vi "While循环的先检查后执行.vi"() -> ()   [LabVIEW 2010]
panel:
  out "温度报警 2":bool
  in  "温度值":dbl(slide) scale=-10.0..10.0
  out "温度报警":bool
  in  "温度值":dbl(slide) scale=-10.0..10.0
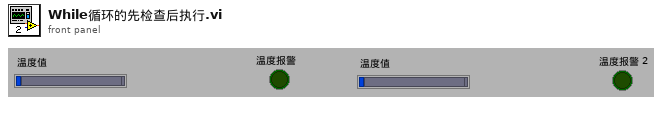
[diagram p1: front panel]
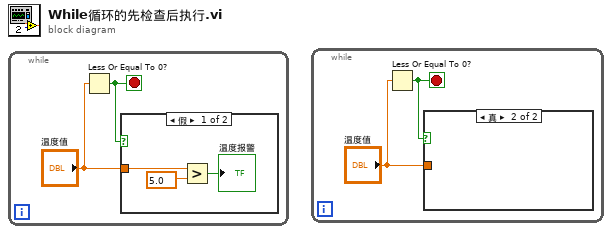
[diagram p0: block diagram]
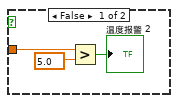
[diagram p2: hidden frame]
diagram:
  n1 = while {
    stop <- w1 stop-if-true
    n2 = Less Or Equal To 0?(x="温度值") -> (x <= 0?=w1:bool)
    n3 = case shown="假" w1 {
      tunnel: "温度值" -> [w4 _]
      frame False {
        n4 = Greater?(x=w4, y=5.0) -> (0:→"温度报警":bool)
      }
      frame True {
      }
    }
  }
  n5 = while {
    stop <- w6 stop-if-true
    n6 = Less Or Equal To 0?(x="温度值") -> (x <= 0?=w6:bool)
    n7 = case shown="真" w6 {
      tunnel: "温度值" -> [w9 _]
      frame False {
        n8 = Greater?(x=w9, y=5.0) -> (0:→"温度报警 2":bool)
      }
      frame True {
      }
    }
  }
